vi "AverageTerminalVoltage.vi"(11 "Raw Terminal Voltage":dbl[][](array[numeric])) -> (3 "Terminal Voltage (MeV)":dbl format="%0.2f")   [LabVIEW 2012]
uses:
  <vilib>/Analysis/baseanly.llb/Mean (DBL).vi
  <vilib>/Analysis/NI_AALBase.lvlib
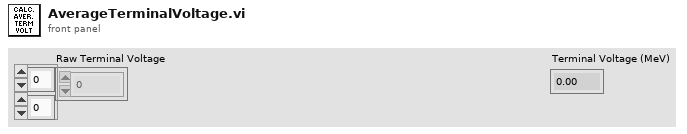
[diagram p1: front panel]
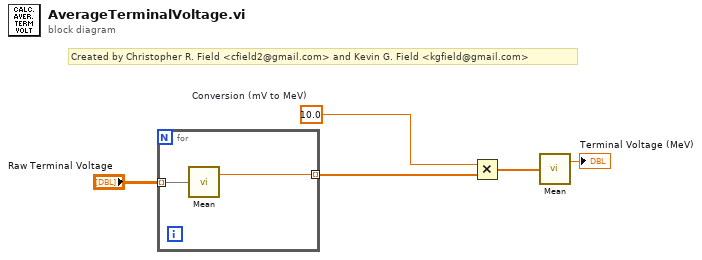
[diagram p0: block diagram]
diagram:
  w4 = 10.0  # Conversion (mV to MeV)
  # "Created by Christopher R. Field <cfield2@gmail.com> and Kevin G. Field <kgfield@gmail.com>"
  n1 = for {
    tunnel: "Raw Terminal Voltage" -> [w7] mode=indexing
    tunnel: [w6] -> w3 mode=indexing
    n2 = call-poly <vilib>:"Mean.vi"("X"=w7) -> ("mean"=w6:dbl)  [unwired: 1 out]
  }
  n3 = Multiply(x=w4, y=w3) -> (x*y=w2:dbl[])
  n4 = call-poly <vilib>:"Mean.vi"("X"=w2) -> ("mean"=→"Terminal Voltage (MeV)":dbl)  [unwired: 1 out]
